vi "UTIL Convert to dB.vi"(1 "Features In":dbl[](array[numeric])) -> (0 "Features (dB)":dbl[](array[numeric]))   [LabVIEW 2017]
doc: "This VI converts a 3-Dimensional feature vector into decibel scale (dB).\n\nInput \n Features In 1-D Array of DBL\nOutput\n Features (dB) 1-D Array of DBL"
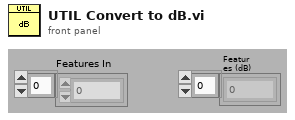
[diagram p1: front panel]
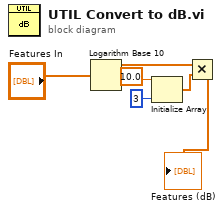
[diagram p0: block diagram]
diagram:
  n1 = Logarithm Base 10(1:"Features In") -> (0:w1:dbl[])
  n2 = Initialize Array(10.0 ("element"), 3 ("dimension size")) -> (w2:dbl[])
  n3 = Multiply(x=w1, y=w2) -> (x*y=→"Features (dB)":dbl[])
